vi "XY Galvo Generator Underscan.v2.vi"(1 "FOV max / V":dbl, 2 "FOV min/ V":dbl, 3 "Microscope Settings in":T1={"Mode"=enum."X", "Slit"={"Scanning Mode"=0.0, "Slit Width /%"=0.0}, "Colour"=[], "Exposure/ms"=0.0, "Piezo Position /um"=0.0, "ROI"={"X"={"Start /px"=0.0, "Step /px"=0.0, "Range /px"=0.0}, "Y"={"Start /px"=0.0, "Step /px"=0.0, "Range /px"=0.0}, "Z "={"Start /um"=0.0, "Step/um"=0.0, "Range /um"=0.0}, "T "={"Start /s"=0.0, "Step /s"=1.0, "Range /s"=100.0}}, "Samples per millisecond"=0.0, "Relax/ms"=0.0, "Readout Direction"=0.0, "Trigger Source"=0.0, "Camera Delay /ms"=0.0, "Under Scan /ms"=0.0, "Waveforms"={"Analogue Out"=[{"t0"=timestamp(0 s since 1904-01-01), "dt"=1.0, "Y"=[]}, {"t0"=timestamp(0 s since 1904-01-01), "dt"=1.0, "Y"=[]}, {"t0"=timestamp(0 s since 1904-01-01), "dt"=1.0, "Y"=[]}], "Digital Out"=[{"t0"=timestamp(0 s since 1904-01-01), "dt"=0.0, "Y"={"transitions"=[], "data"=[]}}, {"t0"=timestamp(0 s since 1904-01-01), "dt"=0.0, "Y"={"transitions"=[], "data"=[]}}, {"t0"=timestamp(0 s since 1904-01-01), "dt"=0.0, "Y"={"transitions"=[], "data"=[]}}]}} {"Under Scan /ms" min=0.0 max=10.0 step=0.05; "ROI"."T"."Range /s" min=0.0 max=10.0 step=0.05; "ROI"."T"."Step /s" min=0.0 max=10.0 step=0.05; "ROI"."T"."Start /s" min=0.0 max=10.0 step=0.05; "ROI"."X"."Range /px" min=0.0 max=10.0 step=0.05; "ROI"."X"."Step /px" min=0.0 max=10.0 step=0.05; "ROI"."X"."Start /px" min=0.0 max=10.0 step=0.05; "ROI"."Y"."Range /px" min=0.0 max=10.0 step=0.05; "ROI"."Y"."Step /px" min=0.0 max=10.0 step=0.05; "ROI"."Y"."Start /px" min=0.0 max=10.0 step=0.05; "ROI"."Z"."Range /um" min=0.0 max=10.0 step=0.05; "ROI"."Z"."Step/um" min=0.0 max=10.0 step=0.05; "ROI"."Z"."Start /um" min=0.0 max=10.0 step=0.05; "Colour"."Colour"."Filter" items=["Empty"=1, ""=2, ""=3, "561"=4, ""=5, "488"=6]; "Camera Delay /ms" min=0.0 max=10.0 step=0.05; "Trigger Source" items=["Internal"=1.0, "External"=2.0]; "Readout Direction" items=["Forward"=1.0, "Backward"=2.0]; "Slit"."Scanning Mode" items=["Full Frame"=1.0, "Slit Scanning"=12.0]; "Piezo Position /um" min=0.0 max=10.0 step=0.05}) -> (0 "XY Galvo":dbl[](graph))   [LabVIEW 2016]
uses:
  controls/Microscope Settings.ctl
  controls/ColourCalibration.ctl
  <vilib>/Analysis/1siggen.llb/Ramp Pattern by Samples.vi
  <vilib>/Analysis/NI_AALBase.lvlib
panel:
  out "Signal":dbl[](array[numeric])
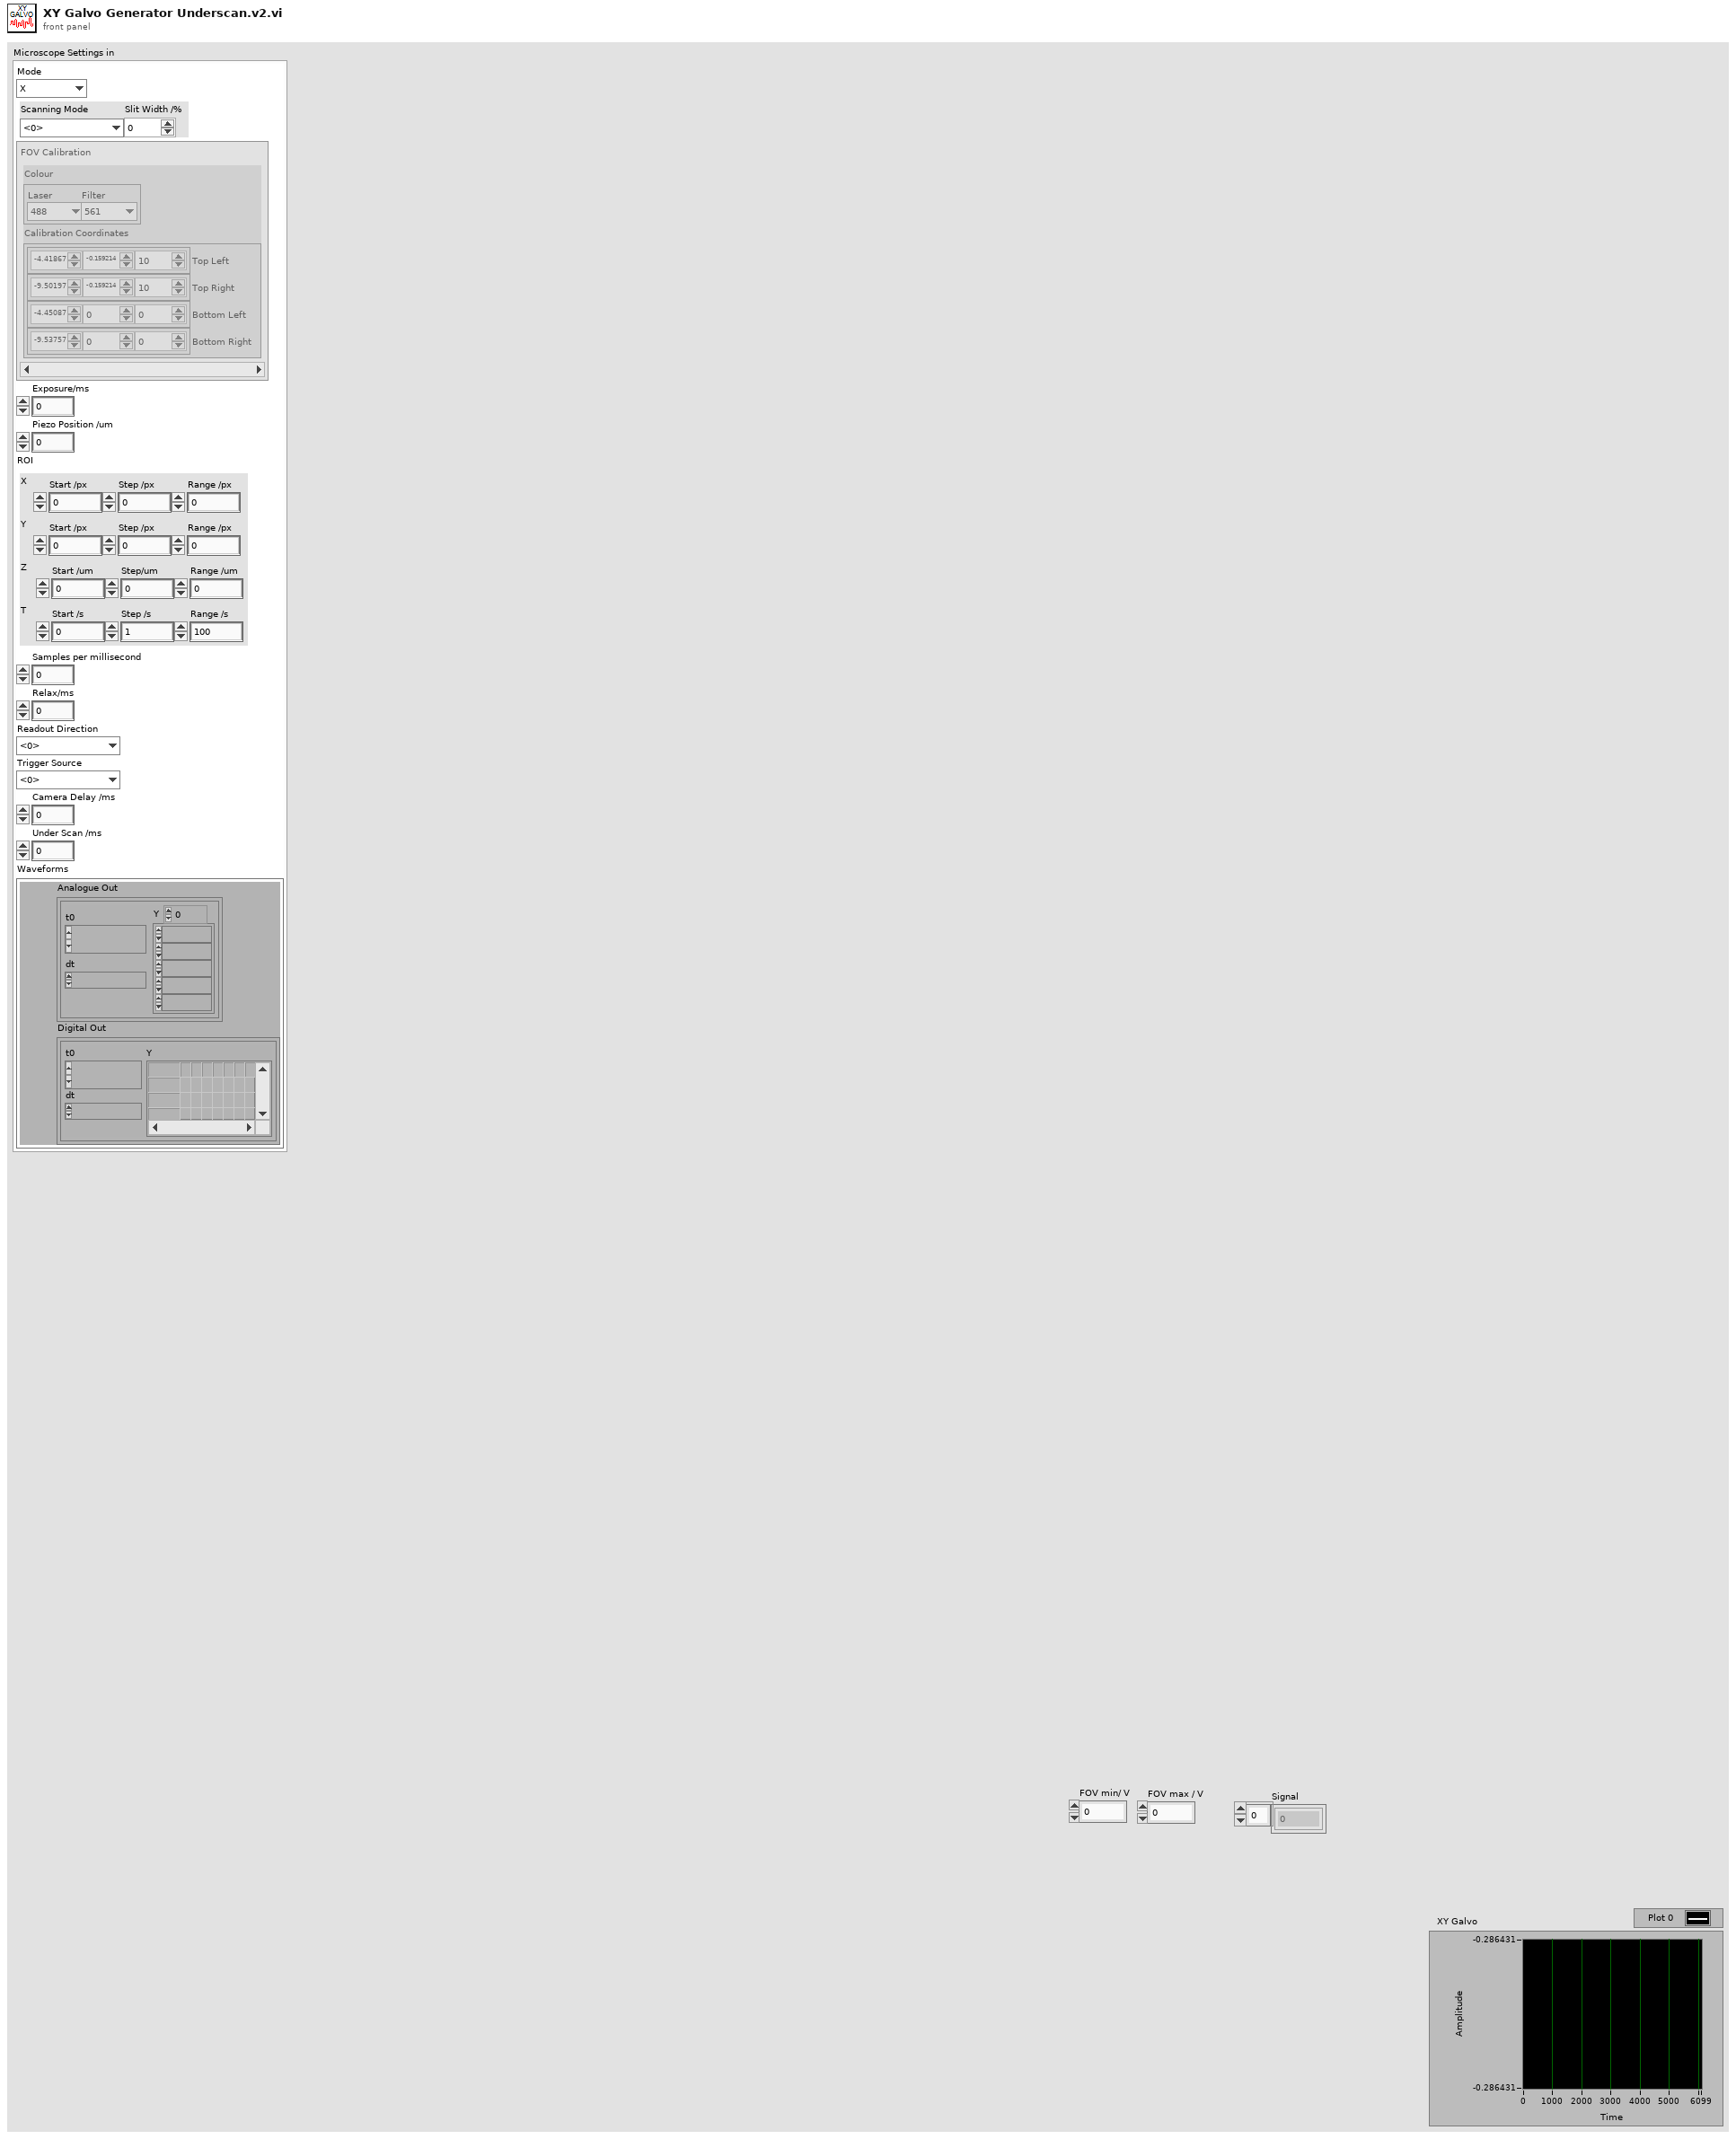
[diagram p1: front panel]
types:
  T1 = typedef "Microscope Settings.ctl" = cluster{"Mode":enum16{"Brightfield", "X", "XY", "XYZ", "XYZT", "XYZC", "Tweezers", "Virus"}, "Slit":cluster{"Scanning Mode":dbl, "Slit Width /%":dbl}, "Colour":T2, "Exposure/ms":dbl, "Piezo Position /um":dbl, "ROI":cluster{"X":cluster{"Start /px":dbl, "Step /px":dbl, "Range /px":dbl}, "Y":cluster{"Start /px":dbl, "Step /px":dbl, "Range /px":dbl}, "Z ":cluster{"Start /um":dbl, "Step/um":dbl, "Range /um":dbl}, "T ":cluster{"Start /s":dbl, "Step /s":dbl, "Range /s":dbl}}, "Samples per millisecond":dbl, "Relax/ms":dbl, "Readout Direction":dbl, "Trigger Source":dbl, "Camera Delay /ms":dbl, "Under Scan /ms":dbl, "Waveforms":cluster{"Analogue Out":waveform(dbl)[], "Digital Out":digitalwaveform[]}}
  T2 = typedef "ColourCalibration.ctl" = cluster{"Colour":cluster{"Laser":enum16{"Brightfield", "445", "488", "561", "647"}, "Filter":u16}, "Calibration Coordinates":cluster{"Top Left":dbl[], "Top Right":dbl[], "Bottom Left":dbl[], "Bottom Right":dbl[]}}[]
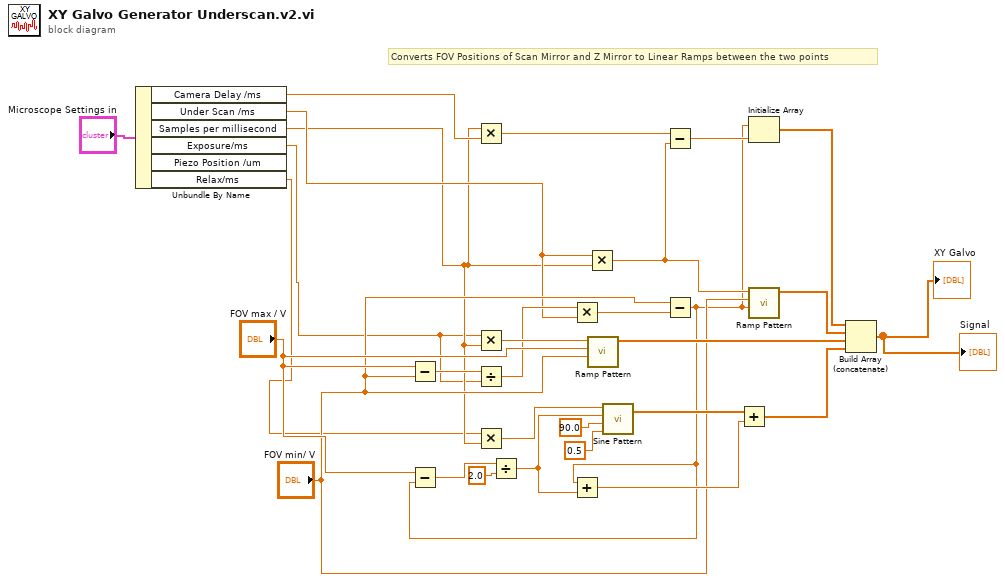
[diagram p0: block diagram]
diagram:
  # "Converts FOV Positions of Scan Mirror and Z Mirror to Linear Ramps between the two points"
  n1 = Unbundle By Name("Microscope Settings in") -> ("Camera Delay /ms"=w5:dbl, "Under Scan /ms"=w4:dbl, "Samples per millisecond"=w3:dbl, "Exposure/ms"=w1:dbl, "Relax/ms"=w2:dbl)  [unwired: 1 out]
  n2 = Subtract(x="FOV max / V", y="FOV min/ V") -> (x-y=w15:dbl)
  n3 = Multiply(x=w3, y=w5) -> (x*y=w14:dbl)
  n4 = Multiply(x=w1, y=w3) -> (x*y=w22:dbl)
  n5 = Divide(x=w15, y=w1) -> (x/y=w17:dbl)
  n6 = Multiply(x=w2, y=w3) -> (x*y=w24:dbl)
  n7 = Multiply(x=w17, y=w4) -> (x*y=w16:dbl)
  n8 = Multiply(x=w4, y=w3) -> (x*y=w13:dbl)
  n9 = call-poly <vilib>:"Ramp Pattern.vi"("start"="FOV min/ V", "end"="FOV max / V", "samples"=w22) -> ("Ramp Pattern"=w10:dbl[])  [unwired: 7 in, 1 out]
  n10 = Subtract(x=w14, y=w13) -> (x-y=w12:dbl)
  n11 = Subtract(x="FOV min/ V", y=w16) -> (x-y=w7:dbl)
  n12 = Subtract(x="FOV max / V", y=w7) -> (x-y=w26:dbl)
  n13 = Divide(x=w26, y=2.0 ("phase(degrees)")) -> (x/y=w29:dbl)
  n14 = Add(x=w7, y=w29) -> (x+y=w28:dbl)
  n15 = call <vilib>:"Sine Pattern.vi"("cycles"=0.5, "phase(degrees)"=90.0, "amplitude"=w29, "samples"=w24) -> ("Sinusoidal Pattern"=w21:dbl[])  [unwired: 1 out]
  n16 = Add(x=w21, y=w28) -> (x+y=w11:dbl[])
  n17 = Initialize Array(w7, w12) -> (w19:dbl[])
  n18 = call-poly <vilib>:"Ramp Pattern.vi"("start"=w7, "end"="FOV min/ V", "samples"=w13) -> ("Ramp Pattern"=w9:dbl[])  [unwired: 7 in, 1 out]
  n19 = Build Array (concatenate)(w19, w9, w10, w11) -> (→"Signal" →"XY Galvo":dbl[])
